vi "pwm_transfer.vi"(7 "pwm method":i32, 8 "tri_wave":fxp<+/-,64,32>, 9 "tri_wave frequency (Hz)":fxp<+,36,20>, 10 "Vdc":fxp<+,12,5>, 11 "signal_input":fxp<+/-,20,5>) -> (2 "pwm_signal":fxp<+/-,20,5>)   [LabVIEW 2014]
uses:
  <vilib>/rvi/Emulation/niFpgaProcessEmulError.vi
panel:
  out "tri_wave time (s)":fxp<+,64,32>
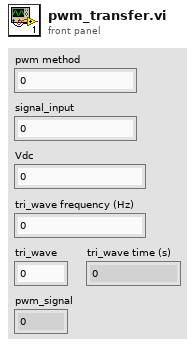
[diagram p1: front panel]
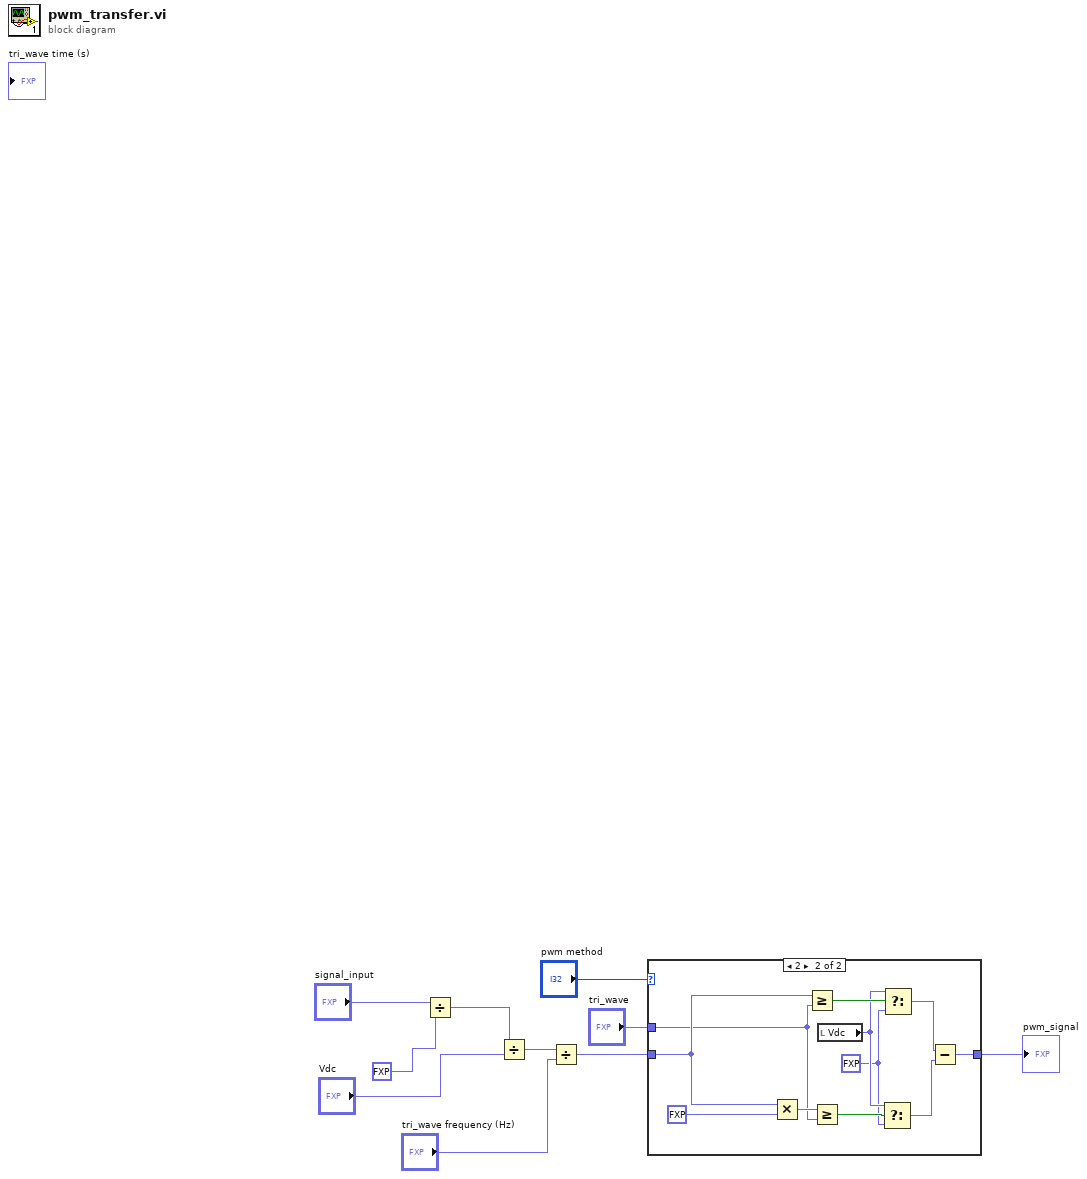
[diagram p0: block diagram]
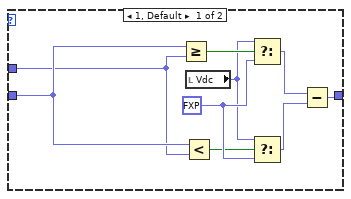
[diagram p2: hidden frame]
diagram:
  n1 = Divide(x="signal_input", y=fxp<+,1,2> 2.0) -> (x/y=w9:fxp<+/-,21,4>)
  n2 = Divide(x=w9, y="Vdc") -> (x/y=w7:fxp<+/-,33,11>)
  n3 = Divide(x=w7, y="tri_wave frequency (Hz)") -> (x/y=w3:fxp<+/-,64,31>)
  n4 = case shown="2" "pwm method" {
    tunnel: w3 -> [w13 w29]
    tunnel: [w11 w21] -> w2
    tunnel: "tri_wave" -> [w12 w20]
    frame 1, Default {
      w19 = fxp<+,12,5> 0.0
      n5 = Greater Or Equal?(x=w13, y=w12) -> (x >= y?=w18:bool)
      n6 = Less?(x=w13, y=w12) -> (x < y?=w17:bool)
      n7 = local read "Vdc"() -> (w14:fxp<+,12,5>)
      n8 = Select(t=w14, s=w18, f=w19) -> (s? t:f=w15:fxp<+,12,5>)
      n9 = Select(t=w14, s=w17, f=w19) -> (s? t:f=w16:fxp<+,12,5>)
      n10 = Subtract(x=w15, y=w16) -> (x-y=w11:fxp<+/-,20,5>)
    }
    frame 2 {
      w24 = fxp<+,12,5> 0.0
      n11 = Multiply(x=w29, y=fxp<+/-,1,1> -1.0) -> (x*y=w27:fxp<+/-,64,33>)
      n12 = Greater Or Equal?(x=w29, y=w20) -> (x >= y?=w30:bool)
      n13 = Greater Or Equal?(x=w27, y=w20) -> (x >= y?=w26:bool)
      n14 = local read "Vdc"() -> (w25:fxp<+,12,5>)
      n15 = Select(t=w25, s=w26, f=w24) -> (s? t:f=w22:fxp<+,12,5>)
      n16 = Select(t=w25, s=w30, f=w24) -> (s? t:f=w23:fxp<+,12,5>)
      n17 = Subtract(x=w23, y=w22) -> (x-y=w21:fxp<+/-,20,5>)
    }
  }
  "pwm_signal" <- w2
